vi "Command_Puke.vi"(0 "Startup":bool, 2 "Timeout":dbl) -> (6 "Reint":bool, 7 "Completed":bool, 8 "Magazine_Velocity":dbl)   [LabVIEW 2020]
uses:
  Auto Utilities/Command_Execution_State.ctl
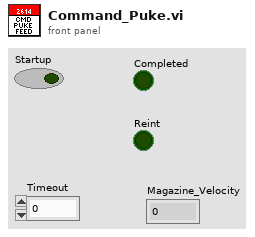
[diagram p1: front panel]
types:
  T1 = typedef "Command_Execution_State.ctl" = enum16{"Initialize", "Execute", "Finish"}
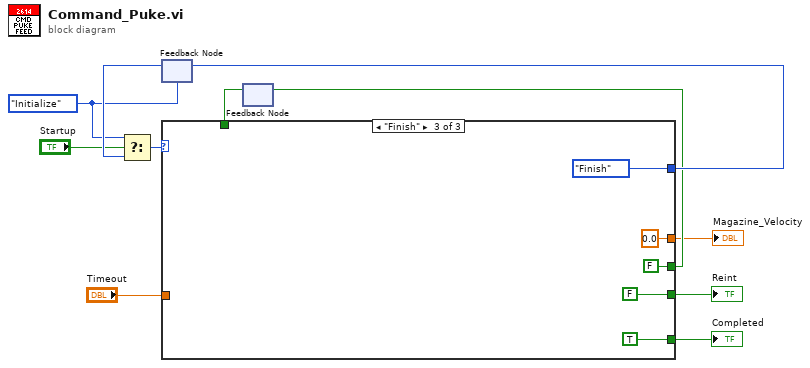
[diagram p0: block diagram]
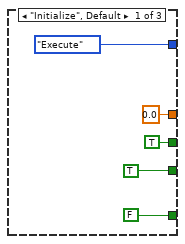
[diagram p2: hidden frame]
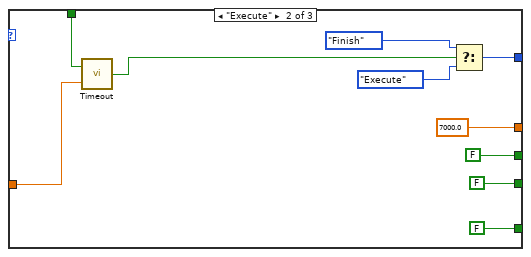
[diagram p3: hidden frame]
diagram:
  w5 = Command_Execution_State."Initialize" ("Play State")
  n1 = feedback #1(w5) -> (w9:T1)
  n2 = Select(t=w5, s="Startup", f=w9) -> (s? t:f=w11:T1)
  n3 = feedback #2() -> (w3:bool)  [unwired: 1 in]
  n4 = case shown="\"Finish\"" w11 {
    tunnel: [Command_Execution_State."Execute" ("Play State") w21 Command_Execution_State."Finish" ("Play State")] -> w10
    tunnel: [FALSE FALSE TRUE] -> w8
    tunnel: [TRUE FALSE FALSE] -> w6
    tunnel: [TRUE FALSE FALSE] -> w4
    tunnel: w3 -> [_ w23 _]
    tunnel: "Timeout" -> [_ w22 _]
    tunnel: [0.0 ("Magazine_Firing_Velocity") 7000.0 ("Magazine_Firing_Velocity") 0.0 ("Magazine_Firing_Velocity")] -> w1
    frame "Initialize", Default {
    }
    frame "Execute" {
      n5 = call "Timeout.vi"("Timeout"=w22, "Initialize"=w23) -> ("Timed Out?"=w18:bool)
      n6 = Select(t=Command_Execution_State."Finish" ("Play State"), s=w18, f=Command_Execution_State."Execute" ("Play State")) -> (s? t:f=w21:T1)
    }
    frame "Finish" {
    }
  }
  "Completed" <- w8
  "Reint" <- w6
  "Magazine_Velocity" <- w1
  n7 = feedback-in #1(w10) -> ()
  n8 = feedback-in #2(w4) -> ()
